vi "CleanUp.vi"(0 "object in":refnum<class "ExtraGUI.lvclass">, 5 "error in (no error)":errorcluster) -> (14 "object out":refnum<class "ExtraGUI.lvclass">, 19 "error out":errorcluster)   [LabVIEW 2017, in "ExtraGUI.lvclass"]
uses:
  ExtraGUI.lvclass
  ExtraGUI.lvclass/ExtraGUI.ctl
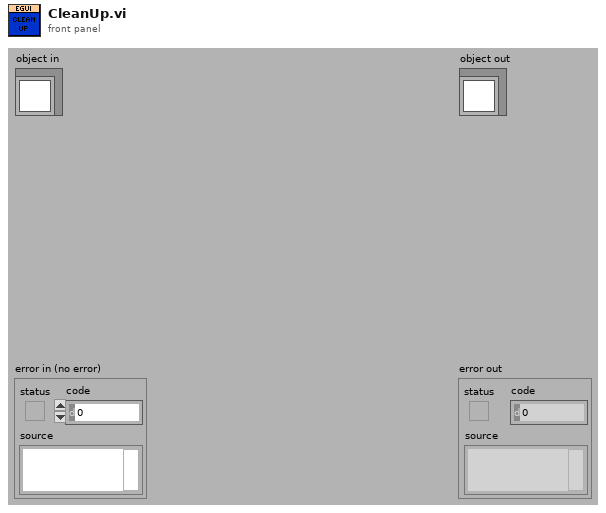
[diagram p1: front panel]
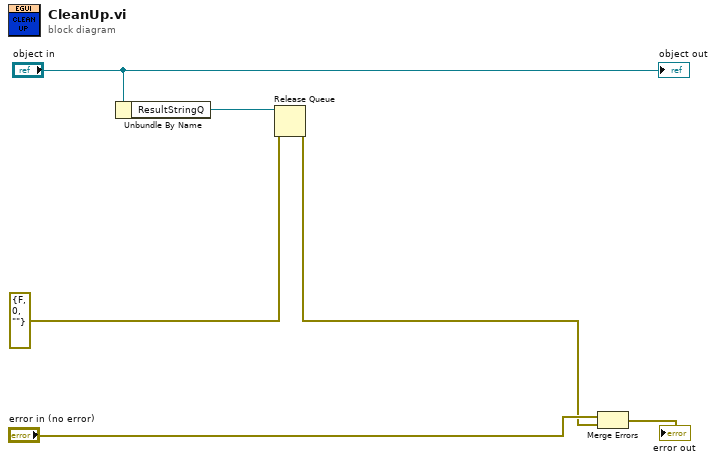
[diagram p0: block diagram]
diagram:
  n1 = Unbundle By Name("object in") -> ("ResultStringQ"=w3:refnum<queue>)
  n2 = Release Queue(queue=w3, error in (no error)=errorcluster {"status"=FALSE, "code"=0, "source"=""}) -> (error out=w1:errorcluster)  [unwired: 1 in, 2 out]
  n3 = Merge Errors("error in (no error)", w1) -> (→"error out":errorcluster)
  "object out" <- "object in"
